vi "Noise Figure Measurement.vi"(6 "Switch":T1, 7 "Path Losses":T2={"DUT Input Loss"={"Compensation Enabled"=1, "Temperation (K)"=297.0, "S2P Path"=path "C:/Users/ies-pg-8881/Desktop/KB/CMT/PS_ATT6dB_26.5GHz.csv", "Orientation"=enum."Port1 Towards DUT"}, "DUT Output Loss"={"Compensation Enabled"=0, "Temperation (K)"=297.0, "S2P Path"=path "C:/Users/ies-pg-8881/Desktop/KB/CMT/PS_ATT6dB_26.5GHz.csv", "Orientation"=enum."Port1 Towards DUT"}, "Calibration Loss"={"Compensation Enabled"=1, "Temperation (K)"=297.0, "S2P Path"=path "C:/Users/ies-pg-8881/Desktop/KB/CMT/PS_ATT6dB_26.5GHz.csv", "Orientation"=enum."Port1 Towards DUT"}, "Noise Source Loss"={"Compensation Enabled"=0, "Temperation (K)"=297.0, "S2P Path"=path "C:/Users/ies-pg-8881/Desktop/KB/CMT/PS_ATT6dB_26.5GHz.csv", "Orientation"=enum."Port1 Towards DUT"}} {"Noise Source Loss"."Compensation Enabled" items=["False", "True"]; "Noise Source Loss"."Temperation (K)" format="%.2g"; "Calibration Loss"."Compensation Enabled" items=["False", "True"]; "Calibration Loss"."Temperation (K)" format="%.2g"; "DUT Output Loss"."Compensation Enabled" items=["False", "True"]; "DUT Output Loss"."Temperation (K)" format="%.2g"; "DUT Input Loss"."Compensation Enabled" items=["False", "True"]; "DUT Input Loss"."Temperation (K)" format="%.2g"}, 8 "error in":errorcluster, 9 "RFmx Settings":T5={"RFmx Name"="5842_0", "RFmx Port"="", "Reference Level"={"DUT Max Gain (dB)"=17.5, "DUT Max Noise Figure (dB)"=3.0, "Mode"=enum."Recommend", "Reference Level (dBm)"=0.0}, "Preamp Enabled"=3, "Attenuation"={"Mode"=enum."Constant Attenuation", "Constant Attenuation"={"RFmx External Attenuation (dB)"=0.8}, "s2p File"={"RFmx S-Parameters Orientation"=24000, "RFmx Attenuation s2p File"=path ""}}, "ENS Source"={"SMU Name"="", "SMU Channel"=""}} {"Attenuation"."s2p File"."RFmx S-Parameters Orientation" items=["Port1 Towards DUT"=24000, "Port2 Towards DUT"=24001]; "Attenuation"."Constant Attenuation"."RFmx External Attenuation (dB)" format="%.2f"; "Preamp Enabled" items=["Disabled"=0, "Enabled"=1, "Automatic"=3]}, 11 "Test Configuration":T4={"Y-Factor Mode"=0, "Measurement Bandwidth (Hz)"=4000000.0, "Measurement Interval (s)"=0.1, "NF Cal Setup ID"="SNS_PS_6dB_ENR15_26.5GHz_VI", "NF DUT Type"=0, "Frequency List (Hz)"=[4000000000.0, 5000000000.0, 6000000000.0, 7000000000.0, 8000000000.0, 9000000000.0, 10000000000.0, 11000000000.0, 12000000000.0, 13000000000.0, 14000000000.0, 15000000000.0, 16000000000.0, 17000000000.0, 18000000000.0, 19000000000.0, 20000000000.0], "Averaging"={"Enabled"=0, "Count"=10}, "Noise Source"={"Noise Source Type"=1, "Noise Source RFSG Port"="", "Cold Temperature (K)"=302.8, "Off Temperature (K)"=297.0, "ENR Freq (Hz)"=[6500000000.0], "ENR (dB)"=[15.0]}} {"Frequency List (Hz)" format="%.3p"; "NF DUT Type" items=["Amplifier", "Downconverter", "Upconverter"]; "Y-Factor Mode" items=["Measure", "Calibrate"]; "Noise Source"."Noise Source Type" items=["External Noise Source", "RF Signal Generator"]; "Noise Source"."ENR (dB)" format="%.2g"; "Noise Source"."ENR Freq (Hz)" format="%.3p"; "Noise Source"."Off Temperature (K)" format="%.2f"; "Noise Source"."Cold Temperature (K)" format="%.2f"; "Averaging"."Enabled" items=["False", "True"]; "Measurement Interval (s)" format="%.2p"; "Measurement Bandwidth (Hz)" format="%.3p"}) -> (0 "error out":errorcluster, 2 "Analyzer Noise Figure (dB)":dbl[][](array[numeric]), 3 "DUT Noise Figure (dB)":dbl[][](array[numeric]), 5 "Results":T6(array[cluster]) {"Frequency (Hz)" format="%.3p"; "Cal Y-Factor (dB)" format="%.2f"; "Meas Y-Factor (dB)" format="%.2f"; "Cold Power (dBm)" format="%.2f"; "Hot Power (dBm)" format="%.2f"; "DUT Gain (dB)" format="%.2f"; "DUT Noise Figure (dB)" format="%.2f"; "DUT Noise Temp (K)" format="%.2f"; "Analyzer Noise Figure (dB)" format="%.2f"})   [LabVIEW 2023]
uses:
  Controls/RFmx Config - NF.ctl
  Controls/Test Config - NF.ctl
  Controls/Path Loss Settings Cluster.ctl
  Controls/Path Loss Settings.ctl
  Controls/Switches - NF.ctl
  <instrlib>/niSwitch/niSwitch.llb/niSwitch Connect Channels (Multiple).vi
panel:
  out "Test Time (ms)":u32
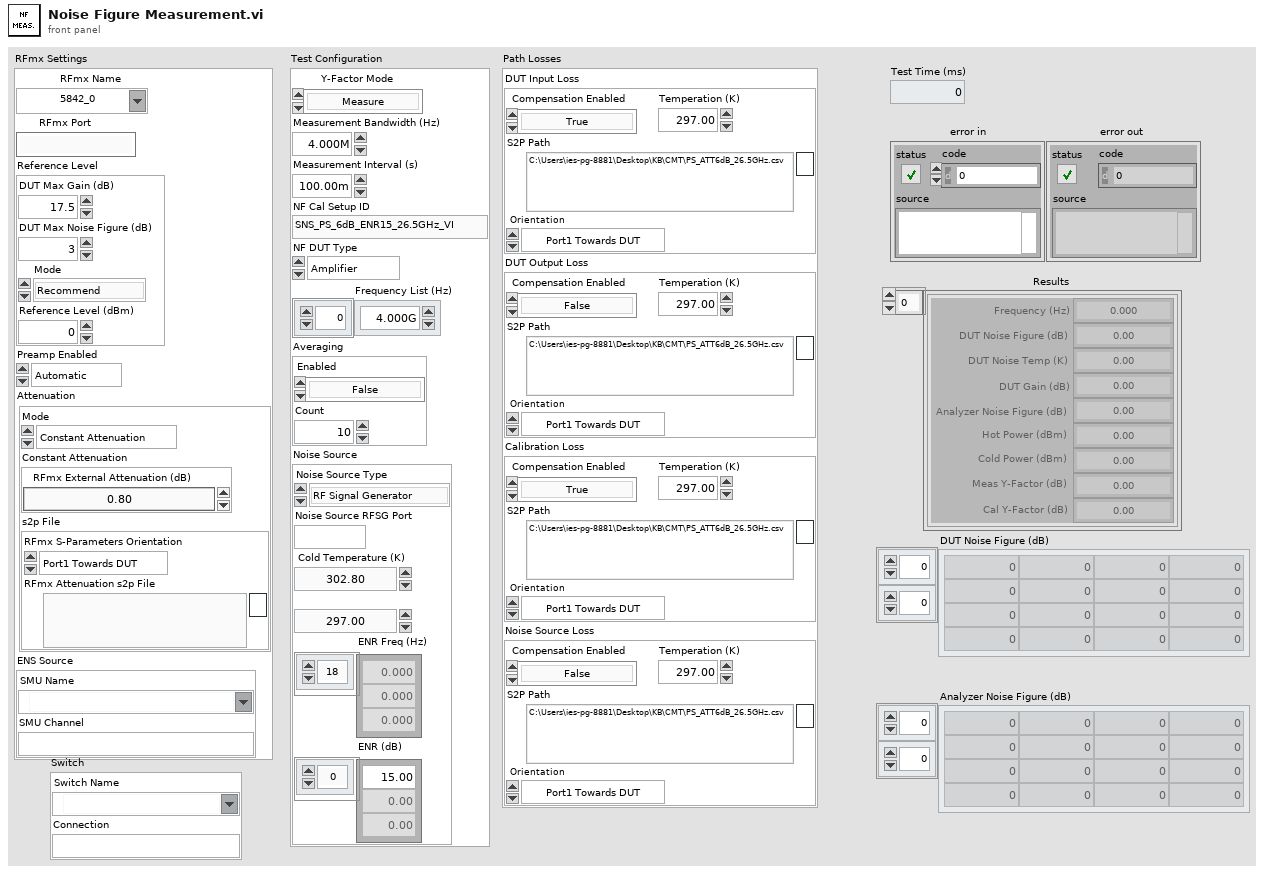
[diagram p1: front panel]
types:
  T1 = typedef "Switches - NF.ctl" = cluster{"Switch Name":refnum<k15>, "Connection":string}
  T2 = typedef "Path Loss Settings Cluster.ctl" = cluster{"DUT Input Loss":T3, "DUT Output Loss":T3, "Calibration Loss":T3, "Noise Source Loss":T3}
  T3 = typedef "Path Loss Settings.ctl" = cluster{"Compensation Enabled":i32, "Temperation (K)":dbl, "S2P Path":path, "Orientation":enum32{"Port1 Towards DUT", "Port2 Towards DUT"}}
  T4 = typedef "Test Config - NF.ctl" = cluster{"Y-Factor Mode":i32, "Measurement Bandwidth (Hz)":dbl, "Measurement Interval (s)":dbl, "NF Cal Setup ID":string, "NF DUT Type":i32, "Frequency List (Hz)":dbl[], "Averaging":cluster{"Enabled":i32, "Count":i32}, "Noise Source":cluster{"Noise Source Type":i32, "Noise Source RFSG Port":string, "Cold Temperature (K)":dbl, "Off Temperature (K)":dbl, "ENR Freq (Hz)":dbl[], "ENR (dB)":dbl[]}}
  T5 = typedef "RFmx Config - NF.ctl" = cluster{"RFmx Name":refnum<k15>, "RFmx Port":string, "Reference Level":cluster{"DUT Max Gain (dB)":dbl, "DUT Max Noise Figure (dB)":dbl, "Mode":enum32{"Manual", "Recommend"}, "Reference Level (dBm)":dbl}, "Preamp Enabled":i32, "Attenuation":cluster{"Mode":enum32{"<None>", "Constant Attenuation", "s2p File"}, "Constant Attenuation":cluster{"RFmx External Attenuation (dB)":dbl}, "s2p File":cluster{"RFmx S-Parameters Orientation":i32, "RFmx Attenuation s2p File":path}}, "ENS Source":cluster{"SMU Name":refnum<k15>, "SMU Channel":string}}
  T6 = cluster{"Frequency (Hz)":dbl, "DUT Noise Figure (dB)":dbl, "DUT Noise Temp (K)":dbl, "DUT Gain (dB)":dbl, "Analyzer Noise Figure (dB)":dbl, "Hot Power (dBm)":dbl, "Cold Power (dBm)":dbl, "Meas Y-Factor (dB)":dbl, "Cal Y-Factor (dB)":dbl}[]
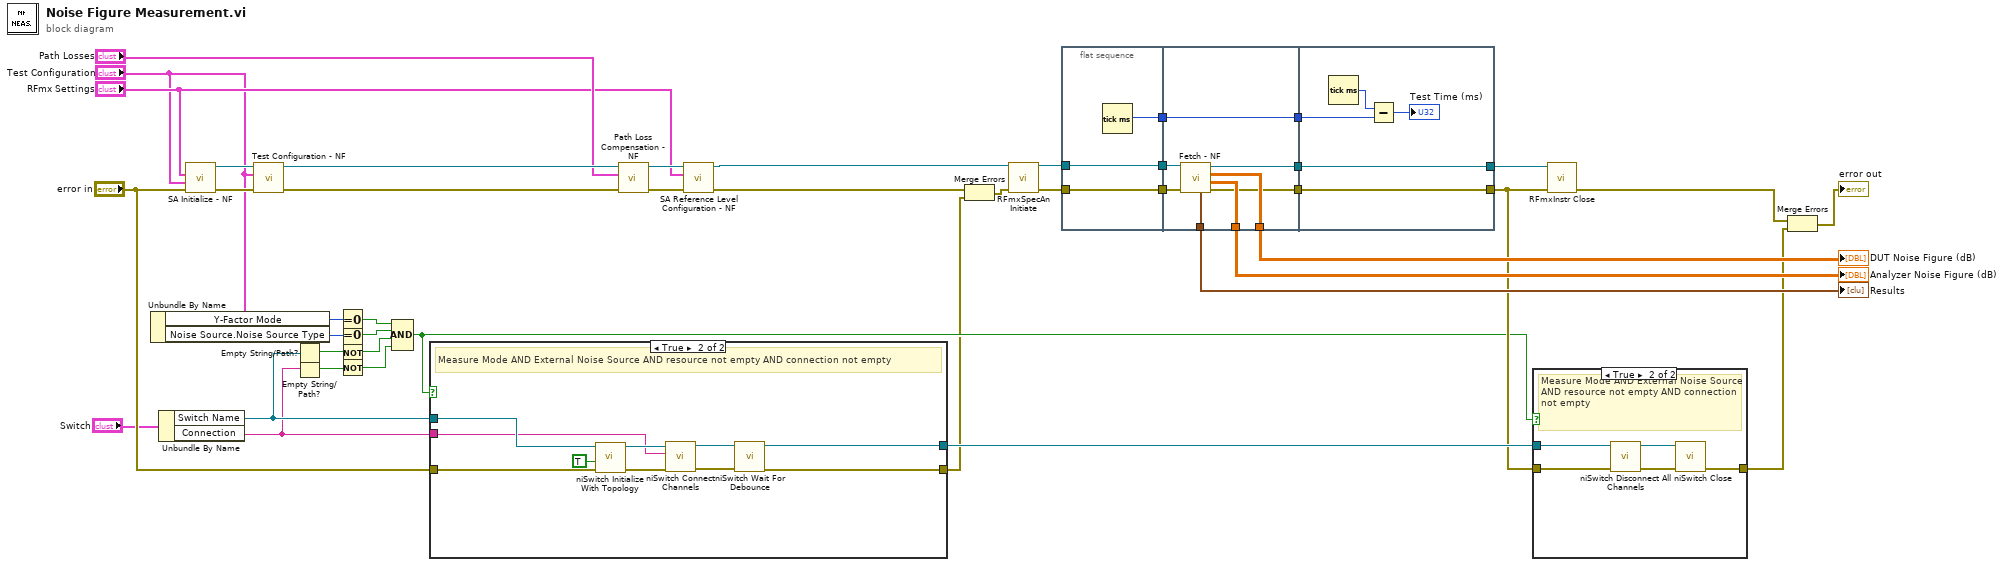
[diagram p0: block diagram]
diagram:
  n1 = Unbundle By Name("Test Configuration") -> ("Y-Factor Mode"=w18:i32, "Noise Source.Noise Source Type"=w17:i32)
  n2 = Unbundle By Name("Switch") -> ("Switch Name"=w4:refnum<k15>, "Connection"=w3:string)
  n3 = call "SA Initialize - NF.vi"("error in"="error in", "Test Configuration"="Test Configuration", "RFmx Settings"="RFmx Settings") -> ("error out"=w39:errorcluster, "RFmx Session out"=w38:refnum<k21>)  [unwired: 7 in]
  n4 = call "Test Configuration - NF.vi"("error in (no error)"=w39, "Test Configuration"="Test Configuration", "RFmx Session in"=w38) -> ("error out"=w8:errorcluster, "RFmx Session out"=w37:refnum<k21>)  [unwired: 7 in]
  n5 = Empty String/Path?(string/path=w4) -> (empty?=w7:bool)
  n6 = Empty String/Path?(string/path=w3) -> (empty?=w6:bool)
  n7 = Equal To 0?(x=w18) -> (x = 0?=w16:bool)
  n8 = Equal To 0?(x=w17) -> (x = 0?=w15:bool)
  n9 = Not(x=w7) -> (.not. x?=w2:bool)
  n10 = Not(x=w6) -> (.not. x?=w1:bool)
  n11 = Compound Arithmetic op=AND(w16, w15, w2, w1) -> (w14:bool)
  n12 = case shown="True" w14 {
    tunnel: "error in" -> [w44 w50]
    tunnel: [w44 w49] -> w9
    tunnel: [_ w47] -> w21
    tunnel: w4 -> [_ w46]
    tunnel: w3 -> [_ w45]
    frame False {
      # "Calibration Mode OR RF Signal Generator"
    }
    frame True {
      # "Measure Mode AND External Noise Source AND resource not empty AND connection not empty"
      n13 = call <instrlib>:"niSwitch Initialize With Topology.vi"("error in (no error)"=w50, "reset device (boolean value)"=TRUE, "resource name"=w46) -> ("error out"=w53:errorcluster, "instrument handle out"=w54:refnum<k15>)  [unwired: 2 in, 5 out]
      n14 = call-poly <instrlib>:"niSwitch Connect Channels.vi"("error in (no error)"=w53, "connection list"=w45, "instrument handle"=w54) -> ("error out"=w51:errorcluster, "instrument handle out"=w52:refnum<k15>)  [unwired: 7 in]
      n15 = call <instrlib>:"niSwitch Wait For Debounce.vi"("error in (no error)"=w51, "instrument handle"=w52) -> ("error out"=w49:errorcluster, "instrument handle out"=w47:refnum<k15>)  [unwired: 1 in, 7 out]
    }
  }
  n16 = call "Path Loss Compensation - NF.vi"("error in (no error)"=w8, "Path Losses"="Path Losses", "RFmx Session in"=w37) -> ("error out"=w26:errorcluster, "RFmx Session out"=w27:refnum<k21>)  [unwired: 7 in]
  n17 = call "SA Reference Level Configuration - NF.vi"("error in"=w26, "RFmx Settings"="RFmx Settings", "RFmx Session in"=w27) -> ("error out"=w25:errorcluster, "RFmx Session out"=w12:refnum<k21>)  [unwired: 7 in]
  n18 = Merge Errors(w25, w9) -> (w10:errorcluster)
  n19 = call <vilib>:"RFmxSpecAn Initiate.vi"("Instrument Handle In"=w12, "error in (no error)"=w10) -> ("Instrument Handle Out"=w42:refnum<k21>, "error out"=w41:errorcluster)  [unwired: 11 in, 1 out]
  n20 = flat-sequence {
    tunnel: w41 -> [w56]
    tunnel: w42 -> [w57]
    tunnel: [w57] -> w35
    tunnel: [w56] -> w34
    tunnel: [w55] -> w31
    tunnel: [w64] -> w28
    tunnel: [w63] -> w29
    tunnel: [w59] -> w40
    tunnel: w35 -> [w61]
    tunnel: w34 -> [w60]
    tunnel: [w65] -> w33
    tunnel: [w62] -> w32
    tunnel: w31 -> [w58]
    tunnel: [w58] -> w30
    tunnel: [w69] -> w20
    tunnel: [w70] -> w43
    tunnel: w33 -> [w70]
    tunnel: w32 -> [w69]
    tunnel: w30 -> [w67]
    frame #0 {
      n21 = Tick Count (ms)() -> (millisecond timer value=w55:u32)
    }
    frame #1 {
      n22 = call "Fetch - NF.vi"("error in"=w60, "Refnum in"=w61) -> ("error out"=w62:errorcluster, "Analyzer Noise Figure (dB)"=w64:dbl[][], "DUT Noise Figure (dB)"=w63:dbl[][], "Refnum out"=w65:refnum<k21>, "Results"=w59:T6)  [unwired: 5 in]
    }
    frame #2 {
      n23 = Tick Count (ms)() -> (millisecond timer value=w68:u32)
      n24 = Subtract(x=w68, y=w67) -> (x-y=→"Test Time (ms)":u32)
    }
  }
  n25 = case shown="True" w14 {
    tunnel: w21 -> [_ w74]
    tunnel: w20 -> [w71 w73]
    tunnel: [w71 w72] -> w19
    frame False {
      # "Calibration Mode OR RF Signal Generator"
    }
    frame True {
      # "Measure Mode AND External Noise Source AND resource not empty AND connection not empty"
      n26 = call <instrlib>:"niSwitch Disconnect All Channels.vi"("error in (no error)"=w73, "instrument handle"=w74) -> ("error out"=w75:errorcluster, "instrument handle out"=w76:refnum<k15>)  [unwired: 8 in]
      n27 = call <instrlib>:"niSwitch Close.vi"("error in (no error)"=w75, "instrument handle"=w76) -> ("error out"=w72:errorcluster)  [unwired: 9 out]
    }
  }
  n28 = call <vilib>:"RFmxInstr Close.vi"("Instrument Handle In"=w43, "error in (no error)"=w20) -> ("error out"=w22:errorcluster)  [unwired: 13 in]
  n29 = Merge Errors(w22, w19) -> (→"error out":errorcluster)
  "Results" <- w40
  "Analyzer Noise Figure (dB)" <- w28
  "DUT Noise Figure (dB)" <- w29
